vi "stabilizePress_07.vi"() -> ()   [LabVIEW 2011]
uses:
  <vilib>/Analysis/NI_AALPro.lvlib
panel:
  in  "max poly order":u16=2
  out "tune setpoint":dbl
  in  "points to fit":i32
  out "dt_array":dbl[](array[numeric])
  out "P_i+1 (torr)":dbl=20.01 caption="predicted next P (torr)" format="%.2f"
  out "Polynomial Coefficients":dbl[](array[numeric])
  in  "polynomial order":dbl
  out "P array":dbl[](array[numeric])
  out "t array":dbl[](array[numeric])
  in  "i":u16
  out "tElaps":dbl=32.29700000002049
  in  "dT_fit(s)":dbl=1.0
  in  "tTotal(s)":dbl=30.0
  out "XY Graph":cluster{"Value":dbl[], "Value":dbl[]}(graph)={"Value"=[1.5420000000158325, 3.0790000000270084, 4.619000000006054, 6.157000000006519, 7.695000000006985, 9.23300000000745, 10.772999999986496, 12.309999999997672, 13.847000000008848, 15.386999999987893, 16.92399999999907, 18.462999999988824, 19.99900000001071, 21.53499999997439, 23.07400000002235, 24.61099999997532, 26.147999999986496, 27.68499999999767, 29.222999999998137, 30.760999999998603, 32.29700000002049], "Value"=[16.36, 19.38, 18.91, 17.669999999999998, 16.93, 17.98, 18.610000000000003, 18.83, 19.259999999999998, 19.459999999999997, 19.55, 19.71, 19.91, 19.939999999999998, 19.92, 19.939999999999998, 19.959999999999997, 19.959999999999997, 19.950000000000003, 19.950000000000003, 20.01]}
  out "stabilize done":bool=TRUE
  in  "tExp(s)":dbl=15.0
  out "Set Point (torr)":dbl=20.0 format="%.2f"
  out "Setpoint Index":string="C"
  out "Setpoint Index control":u16(ring)=2 caption="Setpoint" items=["A", "B", "C", "D"]
  out "t_0":dbl=343263.848
  in  "time done (s)":dbl
  out "Wait to set":bool
  out "IO error":errorcluster={"status"=FALSE, "code"=1073676418, "source"="VISA Close in WriteAdaptorr04.vi->writeSetPoint_01.vi->stabilizePress_05.vi"}
  in  "stop":bool
  out "Pi (torr)":dbl=20.01 caption="P(torr)" format="%.2f"
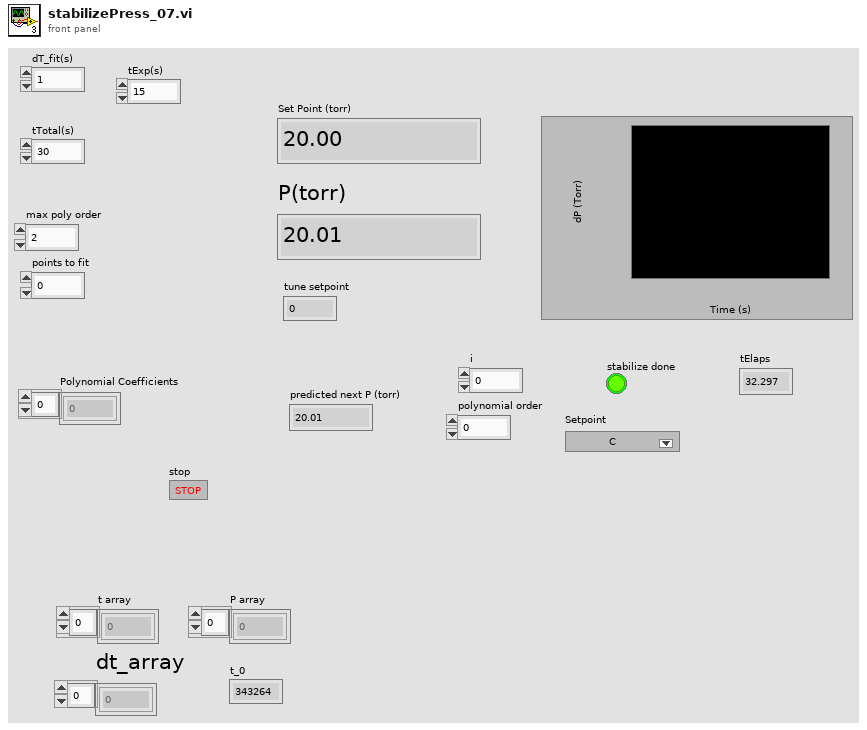
[diagram p1: front panel]
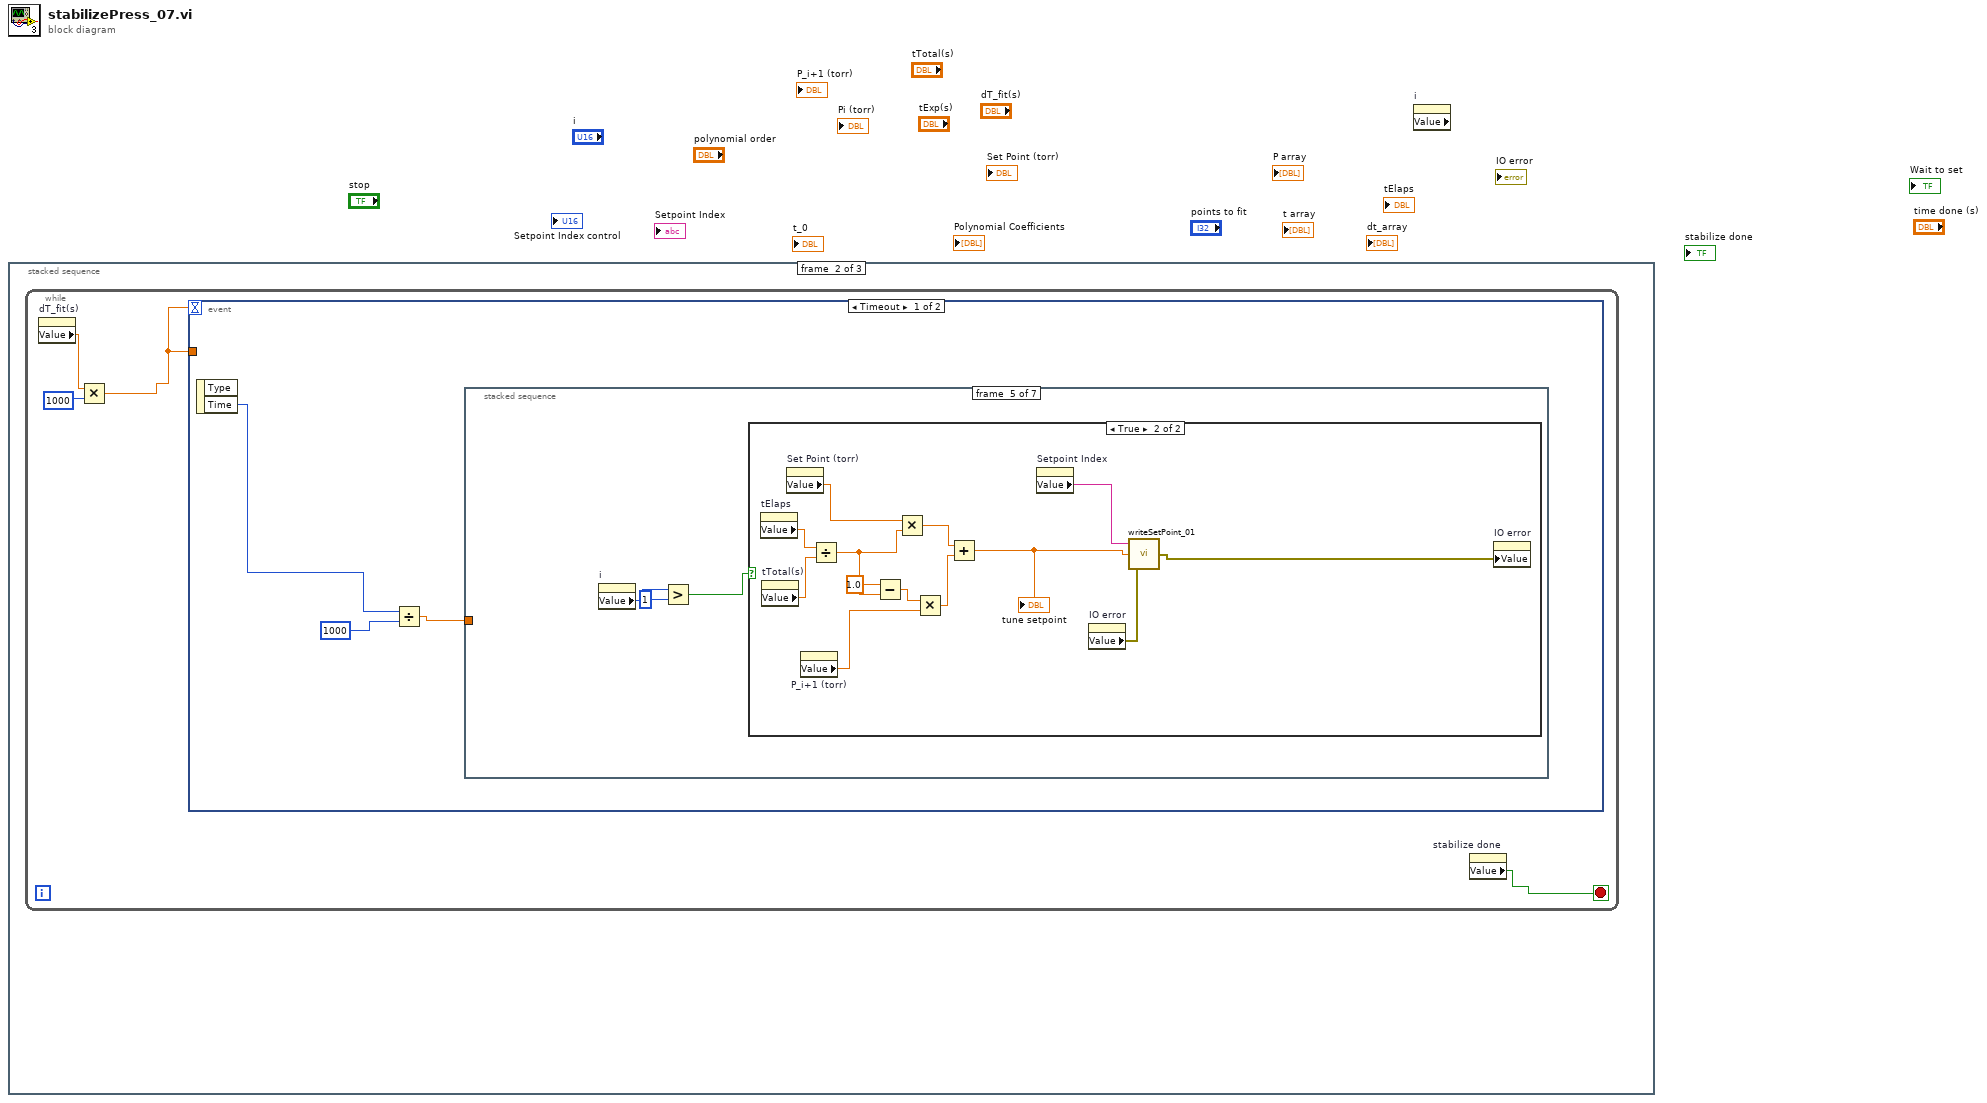
[diagram p0: block diagram]
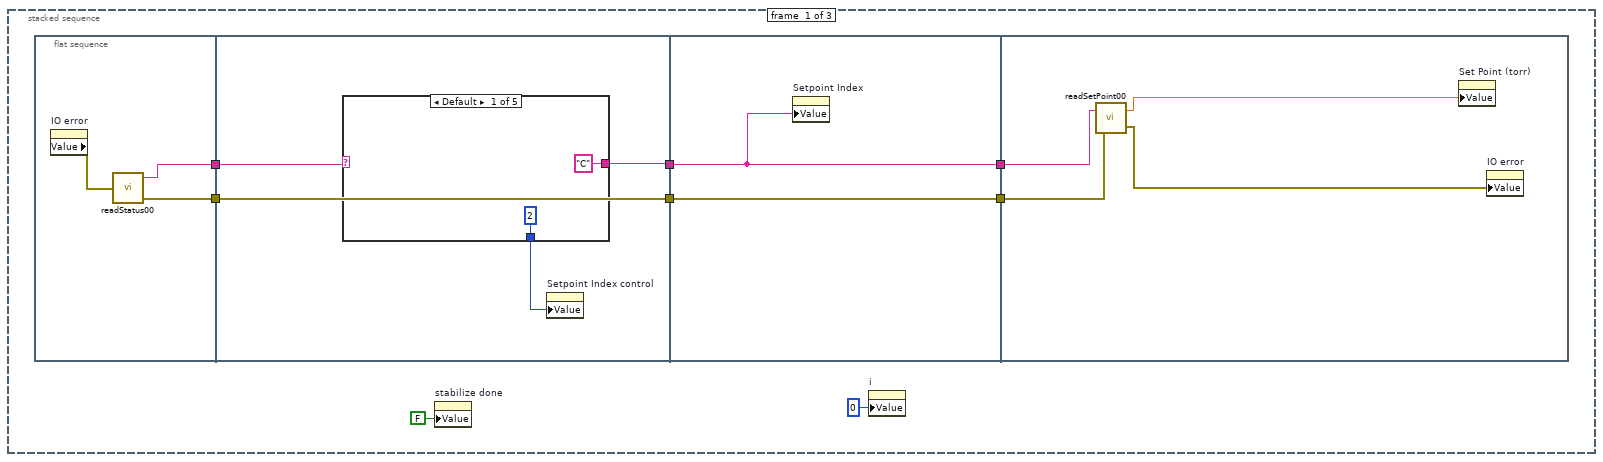
[diagram p2: hidden frame]
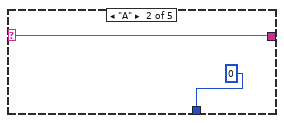
[diagram p3: hidden frame]
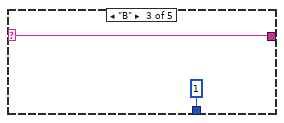
[diagram p4: hidden frame]
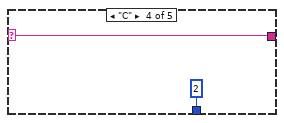
[diagram p5: hidden frame]
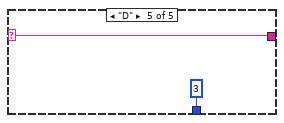
[diagram p6: hidden frame]
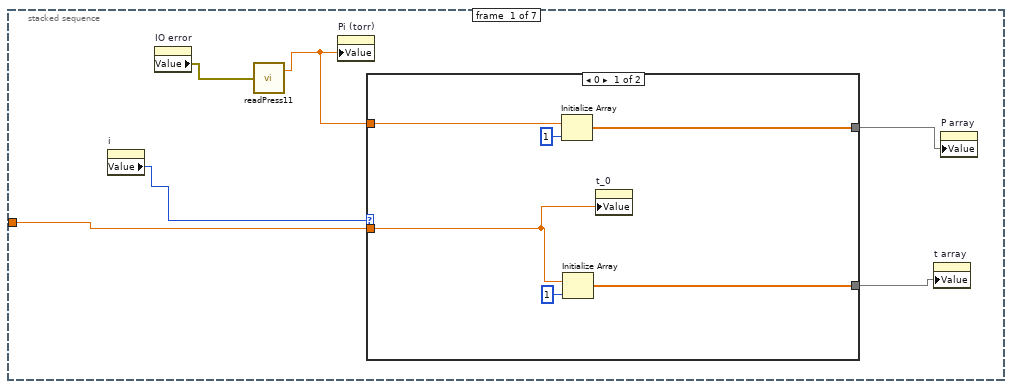
[diagram p7: hidden frame]
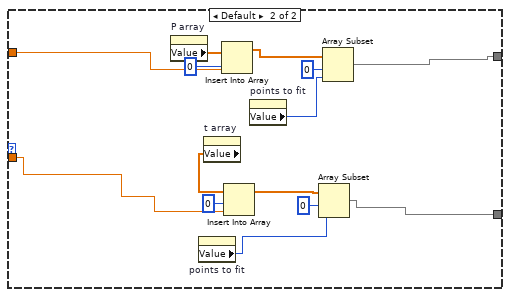
[diagram p8: hidden frame]
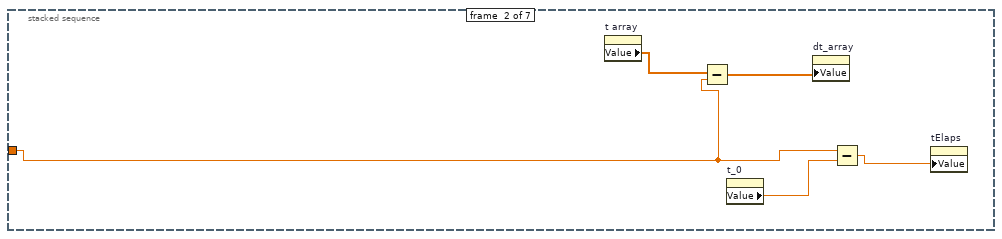
[diagram p9: hidden frame]
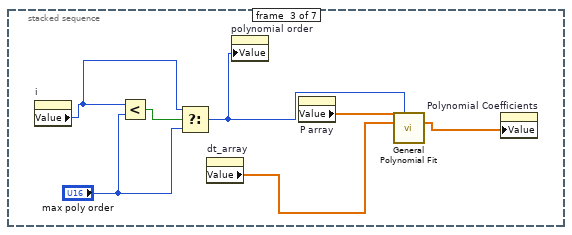
[diagram p10: hidden frame]
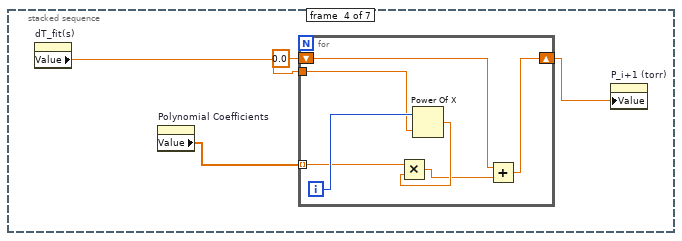
[diagram p11: hidden frame]
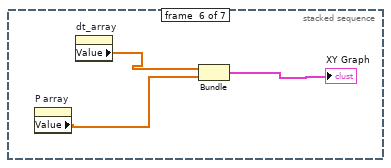
[diagram p13: hidden frame]
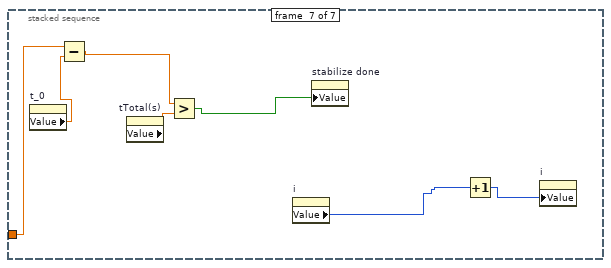
[diagram p14: hidden frame]
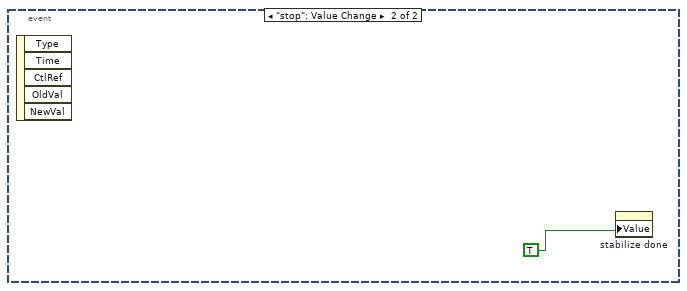
[diagram p15: hidden frame]
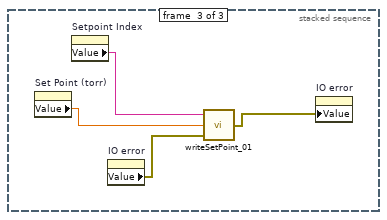
[diagram p16: hidden frame]
diagram:
  n1 = stacked-sequence {
    frame #0 {
      n2 = flat-sequence {
        tunnel: [w10] -> w8
        tunnel: [w9] -> w7
        tunnel: w8 -> [w14]
        tunnel: [w13] -> w6
        tunnel: w7 -> [w15]
        tunnel: [w15] -> w5
        tunnel: w6 -> [w26]
        tunnel: [w26] -> w4
        tunnel: w5 -> [w27]
        tunnel: [w27] -> w3
        tunnel: w4 -> [w31]
        tunnel: w3 -> [w30]
        frame #0 {
          n3 = property on="IO error" class="Clust (strict)"() -> ("Value"=w11:errorcluster)  [unwired: 2 in, 2 out]
          n4 = call "readStatus00.vi"("error in"=w11) -> ("Setpoint"=w10:string, "error out"=w9:errorcluster)  [unwired: 1 out]
        }
        frame #1 {
          n5 = case shown="Default" w14 {
            selector: w14 -> [_ w19 w20 w22 w24]
            tunnel: ["C" w19 w20 w22 w24] -> w13
            tunnel: [u16 2 ("Ring") u16 0 ("Ring") u16 1 ("Ring") u16 2 ("Ring") u16 3 ("Ring")] -> w12
            frame Default {
            }
            frame "A" {
            }
            frame "B" {
            }
            frame "C" {
            }
            frame "D" {
            }
          }
          n6 = property on="Setpoint Index control" class="Ring (strict)"("Value"=w12) -> ()  [unwired: 2 in, 2 out]
        }
        frame #2 {
          n7 = property on="Setpoint Index" class="Str"("Value"=w26) -> ()  [unwired: 2 in, 2 out]
        }
        frame #3 {
          n8 = call "readSetPoint00.vi"("error in"=w30, "Setpoint"=w31) -> ("error out"=w29:errorcluster, "P"=w28:dbl)
          n9 = property on="Set Point (torr)" class="DigNum (strict)"("Value"=w28) -> ()  [unwired: 2 in, 2 out]
          n10 = property on="IO error" class="Clust (strict)"("Value"=w29) -> ()  [unwired: 2 in, 2 out]
        }
      }
      n11 = property on="stabilize done" class="Bool (strict)"("Value"=FALSE ("fit done")) -> ()  [unwired: 2 in, 2 out]
      n12 = property on="i" class="DigNum (strict)"("Value"=u16 0 ("i")) -> ()  [unwired: 2 in, 2 out]
    }
    frame #1 {
      n13 = while {
        stop <- w33 stop-if-true
        n14 = property on="dT_fit(s)" class="DigNum (strict)"() -> ("Value"=w34:dbl)  [unwired: 2 in, 2 out]
        n15 = Multiply(x=w34, y=u32 1000) -> (x*y=w32:dbl)
        n16 = event shown="[0] Timeout" {
          selector: _ -> [_ _]
          dyn-events: _ -> [_ _]
          timeout: w32 -> [_ _]
          tunnel: w32 -> [_ _]
          event Timeout {
            n17 = event-data() -> ("Time"=w36:u32)  [unwired: 1 in, 1 out]
            n18 = Divide(x=w36, y=i64 1000) -> (x/y=w37:dbl)
            n19 = stacked-sequence {
              tunnel: w37 -> [w39 w67 _ _ _ _ w110]
              frame #0 {
                n20 = property on="i" class="DigNum (strict)"() -> ("Value"=w43:u16)  [unwired: 2 in, 2 out]
                n21 = property on="IO error" class="Clust (strict)"() -> ("Value"=w44:errorcluster)  [unwired: 2 in, 2 out]
                n22 = call "readPress11.vi"("error in"=w44) -> ("P"=w42:dbl)  [unwired: 1 out]
                n23 = property on="Pi (torr)" class="DigNum (strict)"("Value"=w42) -> ()  [unwired: 2 in, 2 out]
                n24 = case shown="0" w43 {
                  tunnel: w39 -> [w45 w55]
                  tunnel: w42 -> [w49 w64]
                  tunnel: [w47 w57] -> w41
                  tunnel: [w46 w56] -> w40
                  frame 0 {
                    n25 = Initialize Array(w49, 1 ("dimension size")) -> (w47:dbl[])
                    n26 = Initialize Array(w45, 1 ("dimension size")) -> (w46:dbl[])
                    n27 = property on="t_0" class="DigNum (strict)"("Value"=w45) -> ()  [unwired: 2 in, 2 out]
                  }
                  frame Default {
                    n28 = property on="P array" class="Arr (strict)"() -> ("Value"=w63:dbl[])  [unwired: 2 in, 2 out]
                    n29 = property on="points to fit" class="DigNum (strict)"() -> ("Value"=w51:i32)  [unwired: 2 in, 2 out]
                    n30 = property on="t array" class="Arr (strict)"() -> ("Value"=w62:dbl[])  [unwired: 2 in, 2 out]
                    n31 = Insert Into Array(array=w63, index=0, new element=w64) -> (w61:dbl[])
                    n32 = Insert Into Array(array=w62, index=0, new element=w55) -> (w59:dbl[])
                    n33 = property on="points to fit" class="DigNum (strict)"() -> ("Value"=w52:i32)  [unwired: 2 in, 2 out]
                    n34 = Array Subset(array=w59, index=0, length=w51) -> (w56:dbl[])
                    n35 = Array Subset(array=w61, index=0, length=w52) -> (w57:dbl[])
                  }
                }
                n36 = property on="t array" class="Arr (strict)"("Value"=w40) -> ()  [unwired: 2 in, 2 out]
                n37 = property on="P array" class="Arr (strict)"("Value"=w41) -> ()  [unwired: 2 in, 2 out]
              }
              frame #1 {
                n38 = property on="t array" class="Arr (strict)"() -> ("Value"=w68:dbl[])  [unwired: 2 in, 2 out]
                n39 = Subtract(x=w68, y=w67) -> (x-y=w69:dbl[])
                n40 = property on="t_0" class="DigNum (strict)"() -> ("Value"=w66:dbl)  [unwired: 2 in, 2 out]
                n41 = property on="dt_array" class="Arr (strict)"("Value"=w69) -> ()  [unwired: 2 in, 2 out]
                n42 = Subtract(x=w67, y=w66) -> (x-y=w65:dbl)
                n43 = property on="tElaps" class="DigNum (strict)"("Value"=w65) -> ()  [unwired: 2 in, 2 out]
              }
              frame #2 {
                n44 = property on="i" class="DigNum (strict)"() -> ("Value"=w72:u16)  [unwired: 2 in, 2 out]
                n45 = Less?(x=w72, y="max poly order") -> (x < y?=w75:bool)
                n46 = Select(t=w72, s=w75, f="max poly order") -> (s? t:f=w73:u16)
                n47 = property on="dt_array" class="Arr (strict)"() -> ("Value"=w70:dbl[])  [unwired: 2 in, 2 out]
                n48 = property on="polynomial order" class="DigNum (strict)"("Value"=w73) -> ()  [unwired: 2 in, 2 out]
                n49 = property on="P array" class="Arr (strict)"() -> ("Value"=w76:dbl[])  [unwired: 2 in, 2 out]
                n50 = call <vilib>:"General Polynomial Fit.vi"("Y"=w76, "polynomial order"=w73, "X"=w70) -> ("Polynomial Coefficients"=w74:dbl[])  [unwired: 9 in, 3 out]
                n51 = property on="Polynomial Coefficients" class="Arr (strict)"("Value"=w74) -> ()  [unwired: 2 in, 2 out]
              }
              frame #3 {
                n52 = property on="dT_fit(s)" class="DigNum (strict)"() -> ("Value"=w77:dbl)  [unwired: 2 in, 2 out]
                n53 = property on="Polynomial Coefficients" class="Arr (strict)"() -> ("Value"=w80:dbl[])  [unwired: 2 in, 2 out]
                n54 = for {
                  tunnel: w77 -> [w86]
                  tunnel: w80 -> [w85] mode=indexing
                  shift-right: [w81] -> w78
                  shift-left: 0.0 -> [w82]
                  i -> [w87]
                  n55 = Power Of X(1:w86, 2:w87) -> (0:w84:dbl)
                  n56 = Multiply(x=w85, y=w84) -> (x*y=w83:dbl)
                  n57 = Add(x=w82, y=w83) -> (x+y=w81:dbl)
                }
                n58 = property on="P_i+1 (torr)" class="DigNum (strict)"("Value"=w78) -> ()  [unwired: 2 in, 2 out]
              }
              frame #4 {
                n59 = property on="i" class="DigNum (strict)"() -> ("Value"=w90:u16)  [unwired: 2 in, 2 out]
                n60 = Greater?(x=w90, y=u16 1) -> (0:w88:bool)
                n61 = case shown="True" w88 {
                  frame False {
                  }
                  frame True {
                    n62 = property on="tElaps" class="DigNum (strict)"() -> ("Value"=w100:dbl)  [unwired: 2 in, 2 out]
                    n63 = property on="tTotal(s)" class="DigNum (strict)"() -> ("Value"=w99:dbl)  [unwired: 2 in, 2 out]
                    n64 = property on="Set Point (torr)" class="DigNum (strict)"() -> ("Value"=w98:dbl)  [unwired: 2 in, 2 out]
                    n65 = property on="P_i+1 (torr)" class="DigNum (strict)"() -> ("Value"=w93:dbl)  [unwired: 2 in, 2 out]
                    n66 = Divide(x=w100, y=w99) -> (x/y=w96:dbl)
                    n67 = Subtract(x=1.0, y=w96) -> (x-y=w94:dbl)
                    n68 = Multiply(x=w98, y=w96) -> (x*y=w97:dbl)
                    n69 = Multiply(x=w94, y=w93) -> (x*y=w92:dbl)
                    n70 = Add(x=w97, y=w92) -> (x+y=w91:dbl)
                    "tune setpoint" <- w91
                    n71 = property on="Setpoint Index" class="Str"() -> ("Value"=w103:string)  [unwired: 2 in, 2 out]
                    n72 = property on="IO error" class="Clust (strict)"() -> ("Value"=w102:errorcluster)  [unwired: 2 in, 2 out]
                    n73 = call "writeSetPoint_01.vi"("error in"=w102, "P (Torr)"=w91, "Setpoint"=w103) -> ("error out"=w101:errorcluster)
                    n74 = property on="IO error" class="Clust (strict)"("Value"=w101) -> ()  [unwired: 2 in, 2 out]
                  }
                }
              }
              frame #5 {
                n75 = property on="P array" class="Arr (strict)"() -> ("Value"=w105:dbl[])  [unwired: 2 in, 2 out]
                n76 = property on="dt_array" class="Arr (strict)"() -> ("Value"=w104:dbl[])  [unwired: 2 in, 2 out]
                n77 = Bundle "Bundle"("Value"=w104, "Value"=w105) -> (→"XY Graph":cluster{"Value":dbl[], "Value":dbl[]})  [unwired: 1 in]
              }
              frame #6 {
                n78 = property on="t_0" class="DigNum (strict)"() -> ("Value"=w109:dbl)  [unwired: 2 in, 2 out]
                n79 = Subtract(x=w110, y=w109) -> (x-y=w108:dbl)
                n80 = property on="tTotal(s)" class="DigNum (strict)"() -> ("Value"=w113:dbl)  [unwired: 2 in, 2 out]
                n81 = Greater?(x=w108, y=w113) -> (0:w112:bool)
                n82 = property on="i" class="DigNum (strict)"() -> ("Value"=w107:u16)  [unwired: 2 in, 2 out]
                n83 = property on="stabilize done" class="Bool (strict)"("Value"=w112) -> ()  [unwired: 2 in, 2 out]
                n84 = Increment(x=w107) -> (x+1=w111:u16)
                n85 = property on="i" class="DigNum (strict)"("Value"=w111) -> ()  [unwired: 2 in, 2 out]
              }
            }
          }
          event "stop": Value Change {
            n86 = event-data() -> ()  [unwired: 1 in, 5 out]
            n87 = property on="stabilize done" class="Bool (strict)"("Value"=TRUE ("stabilize done")) -> ()  [unwired: 2 in, 2 out]
          }
        }
        n88 = property on="stabilize done" class="Bool (strict)"() -> ("Value"=w33:bool)  [unwired: 2 in, 2 out]
      }
    }
    frame #2 {
      n89 = property on="Set Point (torr)" class="DigNum (strict)"() -> ("Value"=w118:dbl)  [unwired: 2 in, 2 out]
      n90 = property on="Setpoint Index" class="Str"() -> ("Value"=w117:string)  [unwired: 2 in, 2 out]
      n91 = property on="IO error" class="Clust (strict)"() -> ("Value"=w116:errorcluster)  [unwired: 2 in, 2 out]
      n92 = call "writeSetPoint_01.vi"("error in"=w116, "P (Torr)"=w118, "Setpoint"=w117) -> ("error out"=w115:errorcluster)
      n93 = property on="IO error" class="Clust (strict)"("Value"=w115) -> ()  [unwired: 2 in, 2 out]
    }
  }
  n94 = property on="i" class="DigNum (strict)" props=["Value"]() -> ()  [unwired: 2 in, 3 out]
